vi "SPECTRO.vi"() -> ()   [LabVIEW 2019]
uses:
  Histogram/Histogram.lvlib
  <vilib>/Analysis/NI_AAL_SigProc.lvlib
  <vilib>/Analysis/NI_AALBase.lvlib
panel:
  in  "Tab Control":enum32{"ADC and Decimator", "pAmp CTRL"}(tab)
  in  "Full Scale Range":bool
  in  "DDR":bool
  in  "DCLK_RST":bool
  in  "ON":bool=TRUE
  in  "LED 1":bool
  in  "LED 0":bool=TRUE
  in  "CAL":bool
  in  "CAL_DLY":bool
  in  "OUTV":bool
  out "ADC500_CFG":u32=128
  in  "N":u32=100
  out "number":u32=9
  in  "SET POTS":bool
  in  "FINE OFFSET":u16(slide)=1023 scale=0.0..1023.0
  in  "OFFSET":u16(slide)=1023 scale=0.0..1024.0
  in  "HV_CTRL":bool
  out "RANGE 2":bool=TRUE
  out "RANGE 1":bool
  in  "RANGE":bool
  in  "LED":bool=TRUE
  in  "INIT":bool
  in  "Tab Control 2":T1(tab)
  in  "SET":bool
  in  "TRIGGER_LEVEL":u32=1200
  in  "TRIG_DELAY":u32=500
  in  "FIFO_SIZE":u32=1000
  in  "Trigger Edge":u32(ring)=2 items=["Falling Edge", "Rising Edge", "Auto", "EXT"]
  out "Oscilloscope":waveform(dbl)(graph)
  in  "Store Data":bool caption="Enable"
  in  "CONTINOUS":bool
  in  "Counts":u32
  in  "GEN HISTO":bool
  in  "ENABLE":bool
  out "HISTOGRAM":u32[](graph)
  out "DONE":bool
  out "Progress":u32(slide) max=0
  out "STATUS":u32
  out "pAs_STATUS":u8[](array[numeric])=[1, 0, 0, 0, 9, 0, 0, 0]
  out "PAM_INIT_STATUS":u8[](array[numeric])
  out "ADC500_STATUS":u8[](array[numeric])
  out "DEC_STATUS":u8[](array[numeric])
  in  "address":string="10.47.1.10"
  in  "remote port or service name":u16=7
  out "CONNECTED":bool
  in  "CONNECT":bool
  out "BUSY":bool
  in  "threshold":dbl format="%0.2f"
  in  "width":i32=3 min=3
  in  "initialize (T)":bool=TRUE
  out "# found":i32
  out "Amplitudes":dbl[](array[numeric])
  in  "# bins":i32
  out "Histogram Graph":T2(graph)
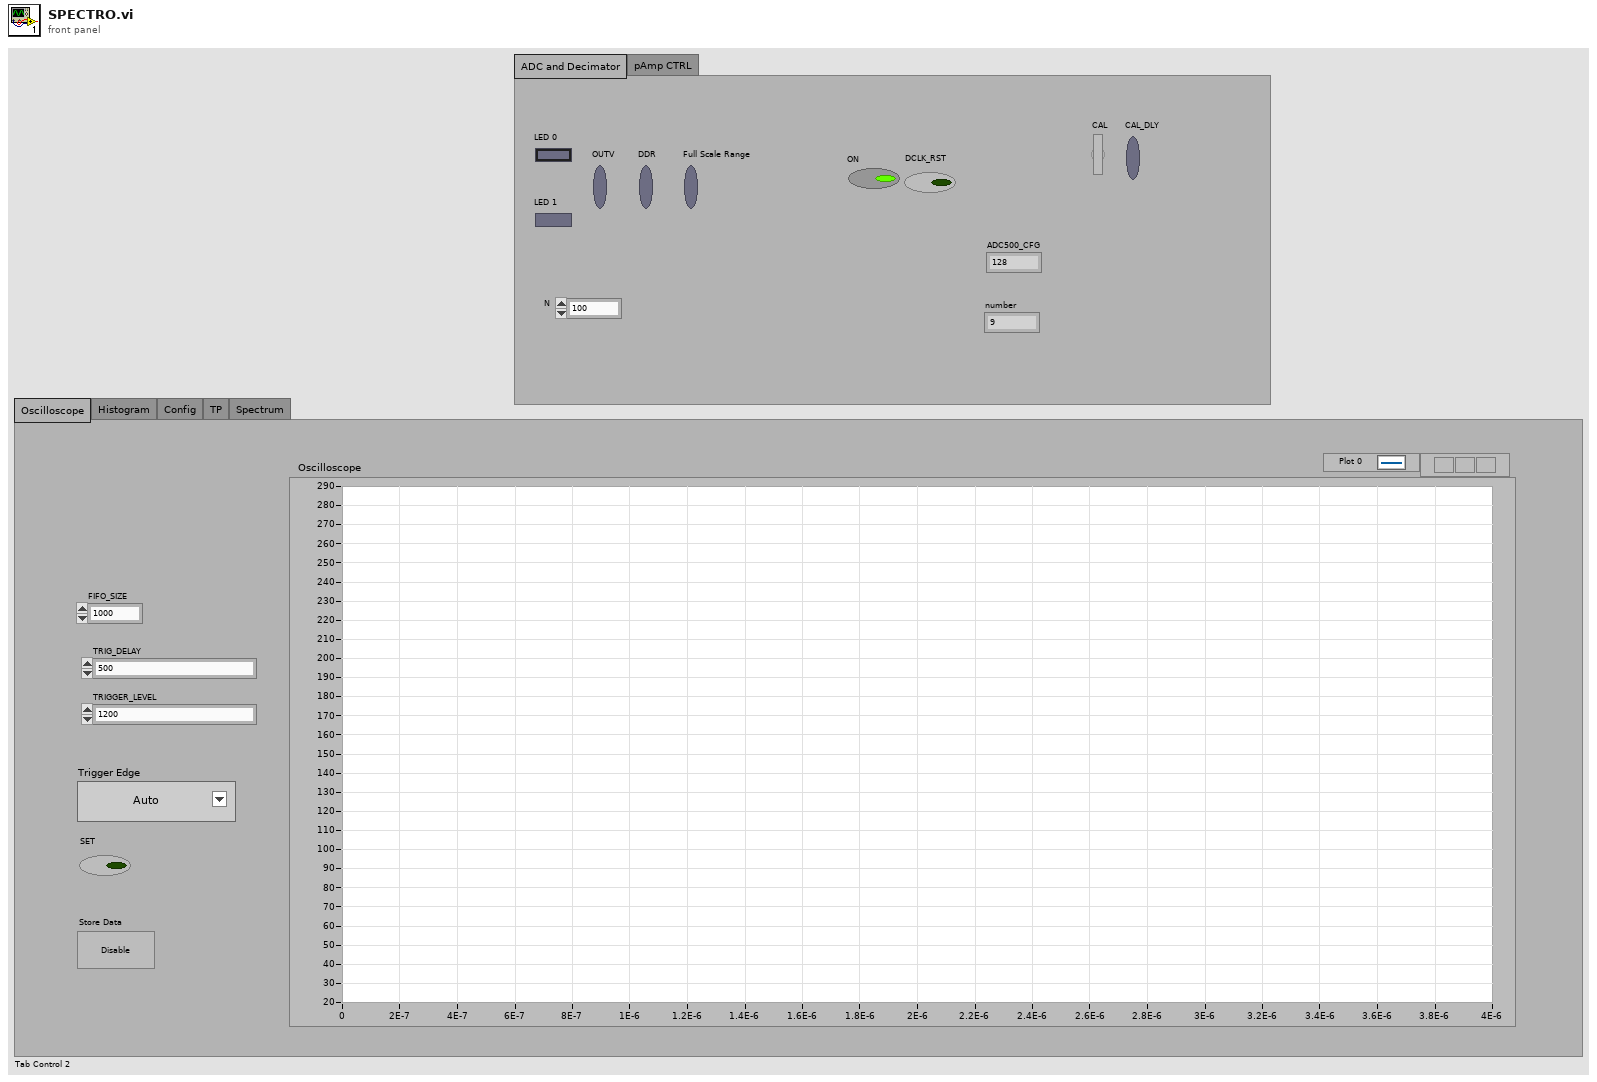
[diagram p1: front panel]
types:
  T1 = enum32{"Oscilloscope", "Histogram", "Config", "TP", "Spectrum"}
  T2 = cluster{"X Values":dbl[], "Histogram: h(x)":i32[]}
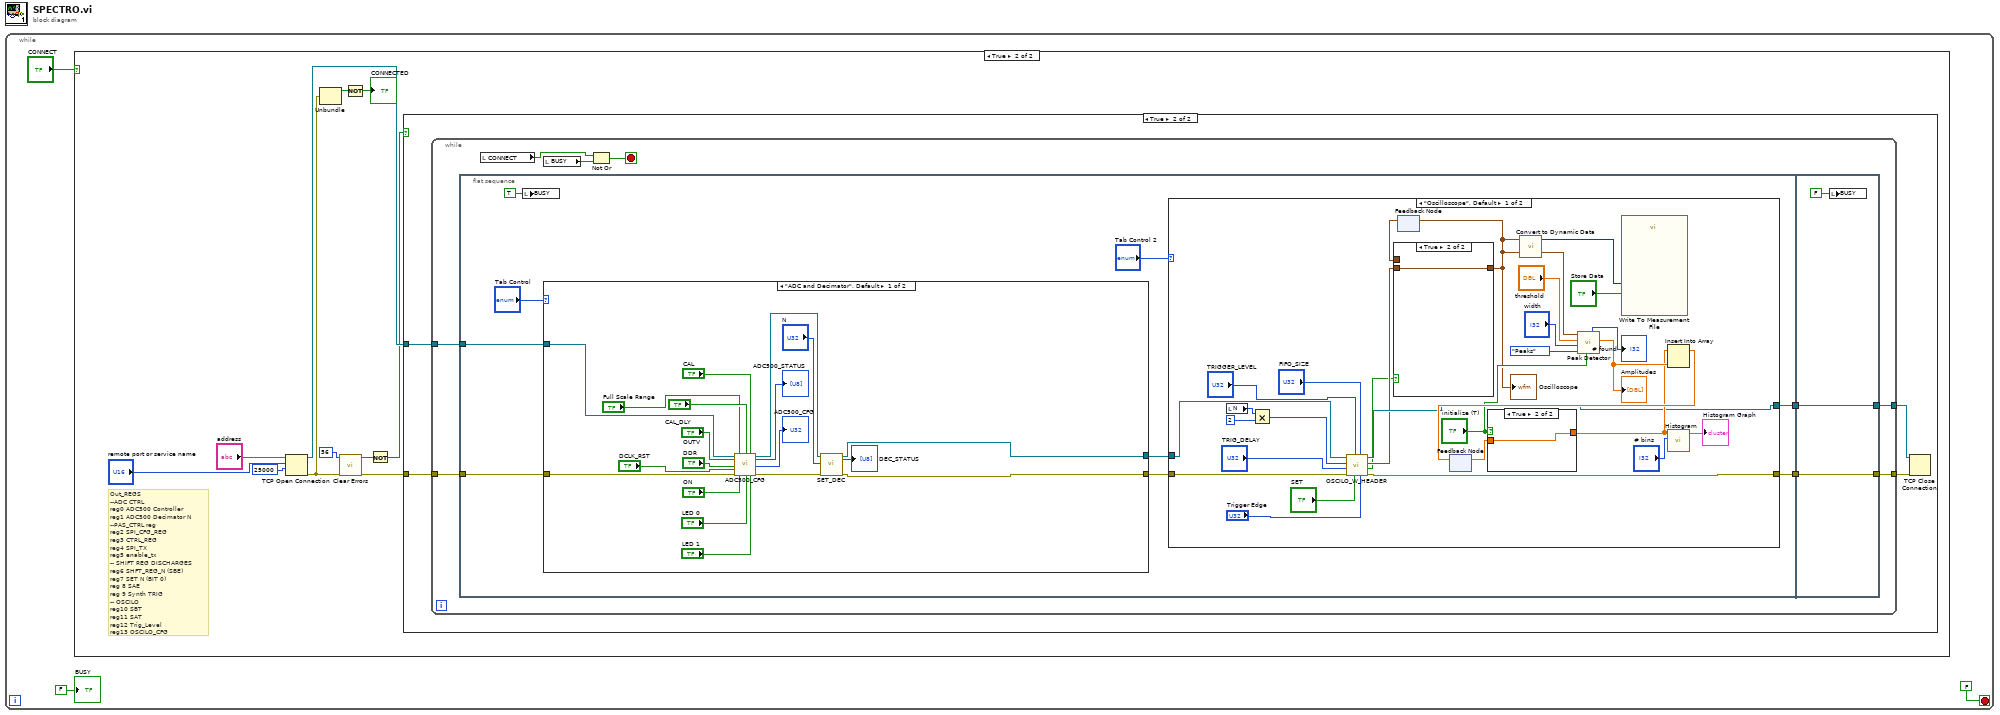
[diagram p0: block diagram]
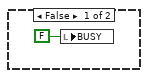
[diagram p3: hidden frame]
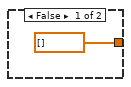
[diagram p5: hidden frame]
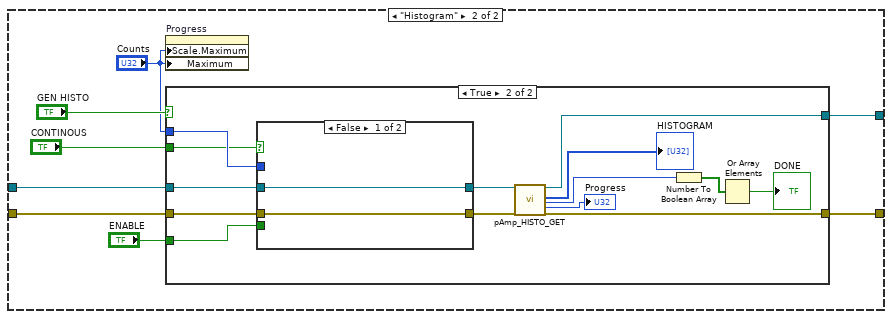
[diagram p6: hidden frame]
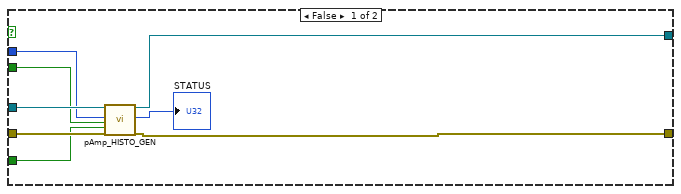
[diagram p7: hidden frame]
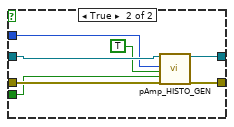
[diagram p8: hidden frame]
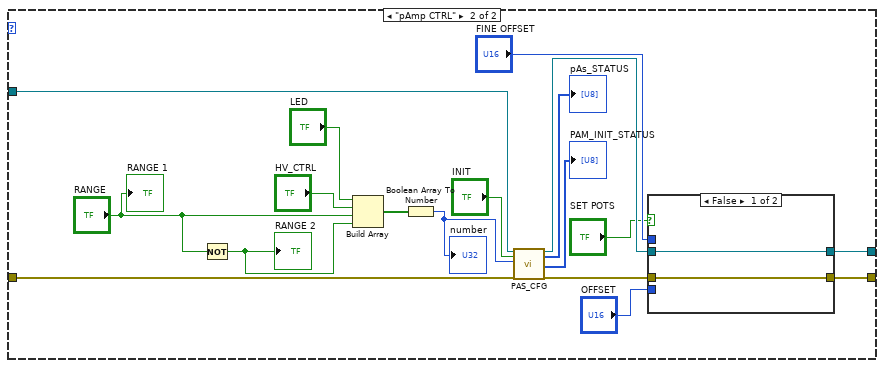
[diagram p9: hidden frame]
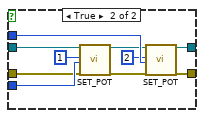
[diagram p10: hidden frame]
diagram:
  n1 = while {
    stop <- FALSE stop-if-true
    n2 = case shown="True" "CONNECT" {
      frame False {
      }
      frame True {
        # "Out_REGS\n--ADC CTRL\nreg0 ADC500 Controller\nreg1 ADC500 Decimator N\n--PAS_CTRL reg\nreg2 SPI_CFG_REG\nreg3 CTRL_REG\nreg4 SPI_TX\nreg5 enable_tx\n-- SHIFT REG DISCHARGES\nreg6 SHFT_REG_N (SBE)\nreg7 SET N (BIT 0)\nreg 8 SAE\nreg 9 Synth TRIG\n-- OSCILO \nreg10 SBT\nreg11 SAT\nreg12 Trig_Level\nreg13 OSCILO_CFG"
        n3 = TCP Open Connection(address="address", remote port or service name="remote port or service name", timeout ms (60000)=25000) -> (connection ID=w14:refnum<k5>, error out=w8:errorcluster)  [unwired: 2 in]
        n4 = Unbundle(w8) -> ("status"=w13:bool)  [unwired: 2 out]
        n5 = call <vilib>:"Clear Errors.vi"("error in (no error)"=w8, "specific error code to clear (0: all)"=56) -> ("error out"=w6:errorcluster, "specific error cleared?"=w5:bool)  [unwired: 4 in]
        n6 = Not(x=w13) -> (.not. x?=→"CONNECTED":bool)
        n7 = Not(x=w5) -> (.not. x?=w4:bool)
        n8 = case shown="True" w4 {
          tunnel: w14 -> [_ w19]
          tunnel: w6 -> [_ w18]
          frame False {
            n9 = local write "BUSY"(FALSE ("BUSY")) -> ()
          }
          frame True {
            n10 = while {
              tunnel: w19 -> [w28]
              tunnel: w18 -> [w27]
              tunnel: [w26] -> w16
              tunnel: [w25] -> w17
              stop <- w20 stop-if-true
              n11 = flat-sequence {
                tunnel: w28 -> [w37]
                tunnel: w27 -> [w36]
                tunnel: [w33] -> w24
                tunnel: [w32] -> w23
                tunnel: [w159] -> w25
                tunnel: [w161] -> w26
                tunnel: w24 -> [w161]
                tunnel: w23 -> [w159]
                frame #0 {
                  n12 = local write "BUSY"(TRUE) -> ()
                  n13 = case shown="\"ADC and Decimator\", Default" "Tab Control" {
                    tunnel: [w112 w132] -> w34
                    tunnel: [w110 w130] -> w30
                    tunnel: w36 -> [w128 w140]
                    tunnel: w37 -> [w127 w141]
                    frame "ADC and Decimator", Default {
                      n14 = call "ADC500_CFG.vi"("TCP Network Connection in"=w127, "OUTV"="OUTV", "DDR"="DDR", "DCLK_RST"="DCLK_RST", "error in (no error)"=w128, "Full Scale Range"="Full Scale Range", "ON"="ON", "CAL_DLY"="CAL_DLY", "LED 0"="LED 0", "CAL"="CAL", "LED 1"="LED 1") -> ("TCP Network Connection out"=w115:refnum<k5>, "ADC500_STATUS"=→"ADC500_STATUS":u8[], "ADC500_CFG"=→"ADC500_CFG":u32, "error out"=w113:errorcluster)  [unwired: 5 in]
                      n15 = call "SET_DEC.vi"("TCP Network Connection in"=w115, "N"="N", "error in (no error)"=w113) -> ("TCP Network Connection out"=w112:refnum<k5>, "DEC_STATUS"=→"DEC_STATUS":u8[], "error out"=w110:errorcluster)  [unwired: 14 in]
                    }
                    frame "pAmp CTRL" {
                      n16 = Not(x="RANGE") -> (.not. x?=w143:bool)
                      "RANGE 2" <- w143
                      n17 = Build Array("LED", "HV_CTRL", "RANGE", w143) -> (w142:bool[])
                      n18 = Boolean Array To Number(Boolean array=w142) -> (number=w139:u32)
                      "number" <- w139
                      n19 = call "PAS_CFG.vi"("TCP Network Connection in"=w141, "INIT"="INIT", "pAs_REG"=w139, "error in (no error)"=w140) -> ("TCP Network Connection out"=w133:refnum<k5>, "pAs_STATUS"=→"pAs_STATUS":u8[], "PAM_INIT"=→"PAM_INIT_STATUS":u8[], "error out"=w131:errorcluster)  [unwired: 12 in]
                      n20 = case shown="False" "SET POTS" {
                        tunnel: "OFFSET" -> [_ w158]
                        tunnel: "FINE OFFSET" -> [_ w157]
                        tunnel: w133 -> [w148 w154]
                        tunnel: [w148 w152] -> w132
                        tunnel: w131 -> [w147 w151]
                        tunnel: [w147 w149] -> w130
                        frame False {
                        }
                        frame True {
                          n21 = call "SET_POT.vi"("TCP Network Connection in"=w154, "POT_N"=u32 1, "VALUE"=w158, "error in (no error)"=w151) -> ("TCP Network Connection out"=w153:refnum<k5>, "error out"=w150:errorcluster)  [unwired: 13 in, 1 out]
                          n22 = call "SET_POT.vi"("TCP Network Connection in"=w153, "POT_N"=u32 2, "VALUE"=w157, "error in (no error)"=w150) -> ("TCP Network Connection out"=w152:refnum<k5>, "error out"=w149:errorcluster)  [unwired: 13 in, 1 out]
                        }
                      }
                      "RANGE 1" <- "RANGE"
                    }
                  }
                  n23 = case shown="\"Oscilloscope\", Default" "Tab Control 2" {
                    tunnel: w34 -> [w53 w78]
                    tunnel: [w48 w76] -> w33
                    tunnel: [w47 w75] -> w32
                    tunnel: w30 -> [w51 w77]
                    frame "Oscilloscope", Default {
                      n24 = local read "N"() -> (w44:u32)
                      n25 = Multiply(x=w44, y=u32 2) -> (x*y=w42:u32)
                      n26 = call "OSCILO_W_HEADER.vi"("Trigger Edge"="Trigger Edge", "FIFO_SIZE"="FIFO_SIZE", "SET"="SET", "TRIGGER_LEVEL"="TRIGGER_LEVEL", "error in (no error)"=w51, "TRIG_DELAY"="TRIG_DELAY", "dt (ns)"=w42, "TCP Network Connection in"=w53) -> ("error out"=w47:errorcluster, "DATA_AVAILABLE"=w38:bool, "output waveform"=w40:waveform(dbl), "TCP Network Connection out"=w48:refnum<k5>)
                      n27 = feedback #1() -> (w41:waveform(dbl))  [unwired: 1 in]
                      n28 = case shown="True" w38 {
                        tunnel: [w67 w68] -> w39
                        tunnel: w40 -> [_ w68]
                        tunnel: w41 -> [w67 _]
                        frame False {
                        }
                        frame True {
                        }
                      }
                      "Oscilloscope" <- w39
                      n29 = feedback-in #1(w39) -> ()
                      n30 = feedback #2() -> (w59:dbl[])  [unwired: 1 in]
                      n31 = case shown="True" "initialize (T)" {
                        tunnel: [dbl[] [] w70] -> w54
                        tunnel: w59 -> [_ w70]
                        frame False {
                        }
                        frame True {
                        }
                      }
                      n32 = call "Convert to Dynamic Data"("Array"=w39) -> ("Dynamic Data Type"=w56:dynamicdata)  [unwired: 3 in]
                      n33 = call <vilib>:"Peak Detector.vi"("initialize (T)"="initialize (T)", "peaks/valleys"=enum32{"Peaks", "Valleys"}."Peaks", "width"="width", "threshold"="threshold", "X"=w39) -> ("Amplitudes"=w61:dbl[], "# found"=→"# found":i32)  [unwired: 2 in, 3 out]
                      "Amplitudes" <- w61
                      n34 = call "Write To Measurement File"("Signals"=w56, "Enable"="Store Data") -> ()  [unwired: 15 in, 3 out]
                      n35 = Insert Into Array(array=w54, new element=w61) -> (w60:dbl[])  [unwired: 1 in]
                      n36 = feedback-in #2(w60) -> ()
                      n37 = call <vilib>:"Histogram.vi"("intervals"="# bins", "X"=w54) -> ("Histogram Graph"=→"Histogram Graph":T2)  [unwired: 6 in, 3 out]
                    }
                    frame "Histogram" {
                      n38 = property on="Progress" class="Slide (strict)"("Scale.Maximum"="Counts", "Maximum"="Counts") -> ()  [unwired: 2 in, 2 out]
                      n39 = case shown="True" "GEN HISTO" {
                        tunnel: w78 -> [w86 w90]
                        tunnel: w77 -> [w85 w91]
                        tunnel: [w80 w95] -> w76
                        tunnel: [w79 w94] -> w75
                        tunnel: "ENABLE" -> [w81 w87]
                        tunnel: "Counts" -> [w84 w89]
                        tunnel: "CONTINOUS" -> [w83 w88]
                        frame False {
                          n40 = call "pAmp_HISTO_GEN.vi"("TCP Network Connection in"=w86, "COUNTS"=w84, "CONTINOUS"=w83, "ENABLE"=w81, "error in (no error)"=w85) -> ("TCP Network Connection out"=w80:refnum<k5>, "STATUS"=→"STATUS":u32, "error out"=w79:errorcluster)  [unwired: 12 in]
                        }
                        frame True {
                          n41 = case shown="False" w88 {
                            tunnel: [w102 w109] -> w93
                            tunnel: [w101 w108] -> w92
                            tunnel: w91 -> [w101 w106]
                            tunnel: w90 -> [w102 w107]
                            tunnel: w89 -> [_ w105]
                            tunnel: w87 -> [_ w103]
                            frame False {
                            }
                            frame True {
                              n42 = call "pAmp_HISTO_GEN.vi"("TCP Network Connection in"=w107, "COUNTS"=w105, "CONTINOUS"=TRUE, "ENABLE"=w103, "error in (no error)"=w106) -> ("TCP Network Connection out"=w109:refnum<k5>, "error out"=w108:errorcluster)  [unwired: 12 in, 1 out]
                            }
                          }
                          n43 = call "pAmp_HISTO_GET.vi"("TCP Network Connection in"=w93, "error in (no error)"=w92) -> ("TCP Network Connection out"=w95:refnum<k5>, "Oscilloscope"=→"HISTOGRAM":u32[], "DONE"=w98:u32, "CURR_COUNT"=→"Progress":u32, "error out"=w94:errorcluster)  [unwired: 12 in, 1 out]
                          n44 = Number To Boolean Array(number=w98) -> (Boolean array=w97:bool[])
                          n45 = Or Array Elements(Boolean array=w97) -> (logical OR=→"DONE":bool)
                        }
                      }
                    }
                  }
                }
                frame #1 {
                  n46 = local write "BUSY"(FALSE) -> ()
                }
              }
              n47 = local read "CONNECT"() -> (w22:bool)
              n48 = local read "BUSY"() -> (w21:bool)
              n49 = Not Or(1:w21, 2:w22) -> (0:w20:bool)
            }
            n50 = TCP Close Connection(connection ID=w16, error in (no error)=w17) -> ()  [unwired: 1 in, 2 out]
          }
        }
      }
    }
    "BUSY" <- FALSE ("BUSY")
  }
